vi "running.set.vi"(10 "running":bool, 11 "manager_daemon in":refnum<class "manager_daemon.lvclass">) -> (3 "manager_daemon out":refnum<class "manager_daemon.lvclass">)   [LabVIEW 2024, in "manager_daemon.lvclass"]
uses:
  manager_daemon.lvclass
  manager_daemon.lvclass/manager_daemon.ctl
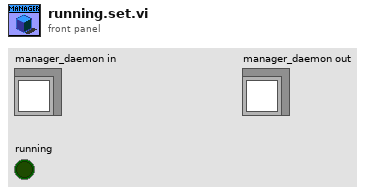
[diagram p1: front panel]
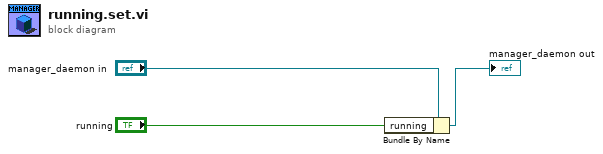
[diagram p0: block diagram]
diagram:
  n1 = Bundle By Name(cluster="manager_daemon in", "running"="running") -> (→"manager_daemon out":refnum<class "manager_daemon.lvclass">)
